vi "Turbulence_1.0.vi"() -> ()   [LabVIEW 2018]
uses:
  <instrlib>/Quantum Composers 9000 Series 2.08/Quantum Composers 9000 Series.lvlib
  <userlib>/LightField Add-in and Automation SDK/Samples/LabVIEW Automation/lightfield-automation-labview/LightField Automation.lvclass
panel:
  in  "Number of Frames":i32
  in  "Intensifier Gain":i32
  in  "Repetitive Gate Width (us)":dbl
  in  "On Chip Accumulations":i32=6
  out "Intensity Graph":dbl[][](graph)
  in  "Experiment Name":string="Experiment1"
  in  "?":bool
  in  "?":bool
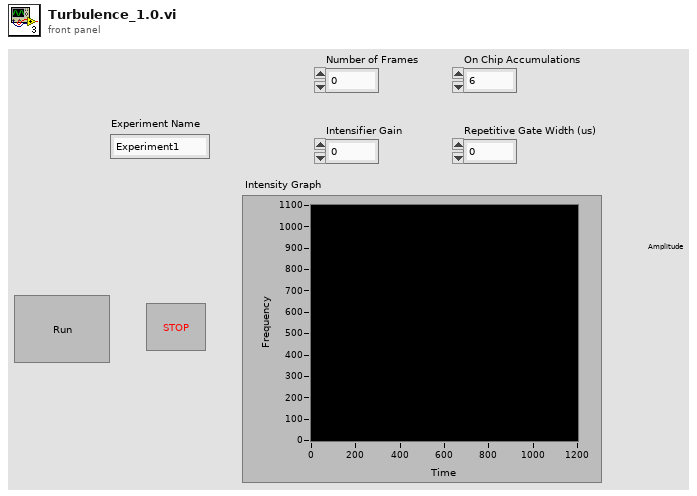
[diagram p1: front panel]
types:
  T1 = cluster{"Image":dbl[][][], "Frame Size":cluster{"F":i32, "Y":i32, "X":i32}}[]
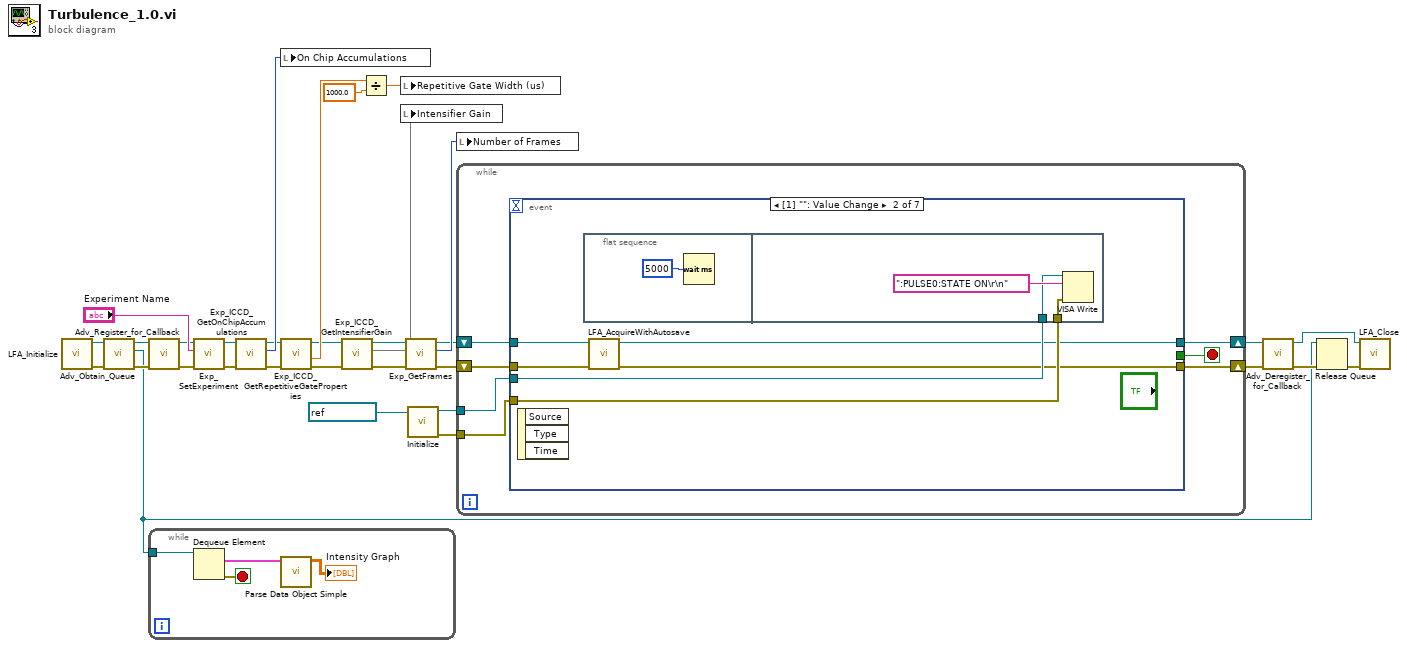
[diagram p0: block diagram]
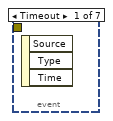
[diagram p2: hidden frame]
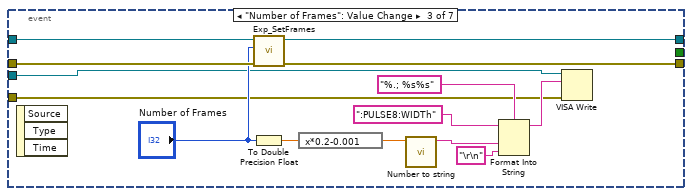
[diagram p3: hidden frame]
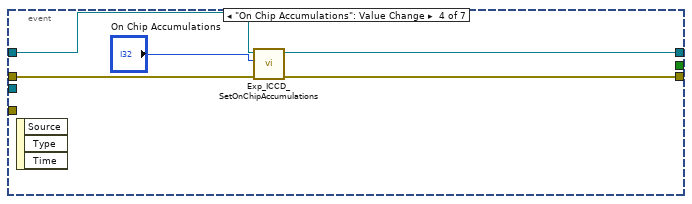
[diagram p4: hidden frame]
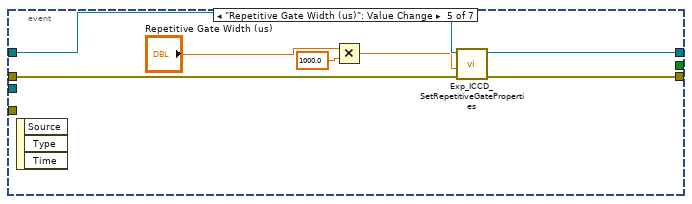
[diagram p5: hidden frame]
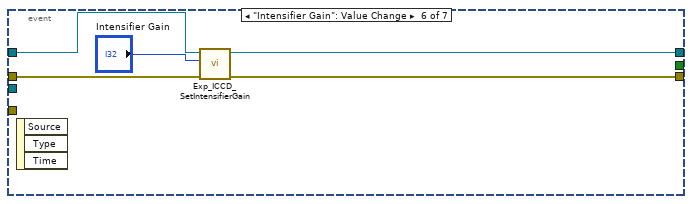
[diagram p6: hidden frame]
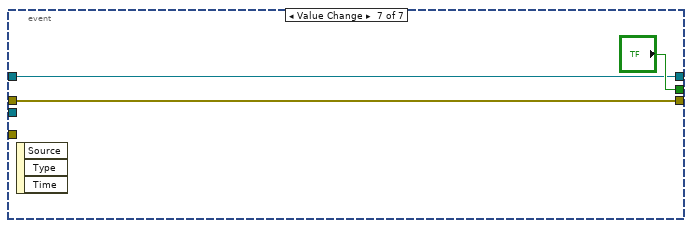
[diagram p7: hidden frame]
diagram:
  n1 = call <userlib>:"LFA_Initialize.vi"() -> ("error out"=w29:errorcluster, "LightField Automation out"=w30:refnum<class "LightField Automation.lvclass">)  [unwired: 10 in]
  n2 = call <userlib>:"Adv_Obtain_Queue.vi"("error in (no error)"=w29, "LightField Automation in"=w30) -> ("error out"=w27:errorcluster, "Queue Reference"=w16:refnum<queue>, "LightField Automation out"=w28:refnum<class "LightField Automation.lvclass">)  [unwired: 7 in]
  n3 = call <userlib>:"Adv_Register_for_Callback.vi"("error in (no error)"=w27, "LightField Automation in"=w28) -> ("error out"=w21:errorcluster, "LightField Automation out"=w22:refnum<class "LightField Automation.lvclass">)  [unwired: 8 in]
  n4 = while {
    tunnel: w16 -> [w36]
    stop <- w35 stop-if-true
    n5 = Dequeue Element(queue=w36) -> (element=w34:T1, error out=w35:errorcluster)  [unwired: 2 in, 2 out]
    n6 = call <userlib>:"Parse Data Object Simple.vi"("Data"=w34) -> ("ROI 1, Frame 1"=→"Intensity Graph":dbl[][])  [unwired: 9 in, 1 out]
  }
  n7 = call <userlib>:"Exp_SetExperiment.vi"("error in (no error)"=w21, "ExperimentName"="Experiment Name", "LightField Automation in"=w22) -> ("error out"=w17:errorcluster, "LightField Automation out"=w18:refnum<class "LightField Automation.lvclass">)  [unwired: 7 in]
  n8 = call <userlib>:"Exp_ICCD_GetOnChipAccumulations.vi"("error in (no error)"=w17, "LightField Automation in"=w18) -> ("error out"=w13:errorcluster, "On Chip Accumulations"=w15:i32, "LightField Automation out"=w14:refnum<class "LightField Automation.lvclass">)  [unwired: 7 in]
  n9 = local write "On Chip Accumulations"(w15) -> ()
  n10 = call <userlib>:"Exp_ICCD_GetRepetitiveGateProperties.vi"("error in (no error)"=w13, "LightField Automation in"=w14) -> ("error out"=w8:errorcluster, "Repetitive Gate Width (ns)"=w12:dbl, "LightField Automation out"=w9:refnum<class "LightField Automation.lvclass">)  [unwired: 6 in, 1 out]
  n11 = call <userlib>:"Exp_ICCD_GetIntensifierGain.vi"("error in (no error)"=w8, "LightField Automation in"=w9) -> ("error out"=w5:errorcluster, 2:w1, "LightField Automation out"=w6:refnum<class "LightField Automation.lvclass">)  [unwired: 6 in, 1 out]
  n12 = Divide(x=w12, y=1000.0) -> (x/y=w10:dbl)
  n13 = local write "Repetitive Gate Width (us)"(w10) -> ()
  n14 = local write "Intensifier Gain"(w1) -> ()
  n15 = call <userlib>:"Exp_GetFrames.vi"("error in (no error)"=w5, "LightField Automation in"=w6) -> ("error out"=w4:errorcluster, "Frames"=w7:i32, "LightField Automation out"=w3:refnum<class "LightField Automation.lvclass">)  [unwired: 7 in]
  n16 = call <instrlib>:"Initialize.vi"("VISA resource name"=refnum<visa-resource-name> "COM16") -> ("error out"=w31:errorcluster, "VISA resource name out"=w32:refnum<visa-resource-name>)  [unwired: 9 in]
  n17 = local write "Number of Frames"(w7) -> ()
  n18 = while {
    tunnel: w32 -> [w42]
    tunnel: w31 -> [w43]
    shift-right: [w40] -> w20
    shift-left: w3 -> [w38]
    shift-right: [w41] -> w19
    shift-left: w4 -> [w39]
    stop <- w37 stop-if-true
    n19 = event shown="[1] \"\": Value Change" {
      selector: _ -> [_ _ _ _ _ _ _]
      dyn-events: _ -> [_ _ _ _ _ _ _]
      timeout: _ -> [_ _ _ _ _ _ _]
      tunnel: w43 -> [_ w49 w57 _ _ _ _]
      tunnel: w42 -> [_ w48 w58 _ _ _ _]
      tunnel: w39 -> [_ w47 w64 w71 w78 w82 w85]
      tunnel: w38 -> [_ w46 w67 w72 w79 w83 w86]
      tunnel: [_ w45 w65 w69 w76 w80 w85] -> w41
      tunnel: [_ w44 w66 w70 w77 w81 w86] -> w40
      tunnel: [_ _ _ _ _ _ "?"] -> w37
      event Timeout {
        n20 = event-data() -> ()  [unwired: 1 in, 3 out]
      }
      event Value Change {
        n21 = event-data() -> ()  [unwired: 1 in, 3 out]
        n22 = flat-sequence {
          tunnel: w49 -> [w53]
          tunnel: w48 -> [w51]
          frame #0 {
            n23 = Wait (ms)(milliseconds to wait=5000) -> ()  [unwired: 1 out]
          }
          frame #1 {
            n24 = VISA Write(VISA resource name=w51, write buffer=":PULSE0:STATE ON\r\n" ("format string"), error in (no error)=w53) -> ()  [unwired: 3 out]
          }
        }
        n25 = call <userlib>:"LFA_AcquireWithAutosave.vi"("error in (no error)"=w47, "LightField Automation in"=w46) -> ("error out"=w45:errorcluster, "LightField Automation out"=w44:refnum<class "LightField Automation.lvclass">)  [unwired: 7 in, 1 out]
      }
      event "Number of Frames": Value Change {
        n26 = event-data() -> ()  [unwired: 1 in, 3 out]
        n27 = call <userlib>:"Exp_SetFrames.vi"("error in (no error)"=w64, "Number of Frames"="Number of Frames", "LightField Automation in"=w67) -> ("error out"=w65:errorcluster, "LightField Automation out"=w66:refnum<class "LightField Automation.lvclass">)  [unwired: 7 in]
        n28 = To Double Precision Float(number="Number of Frames") -> (double precision float=w62:dbl)
        n29 = expression code="x*0.2-0.001"(w62) -> (w56:dbl)
        n30 = call "Number to string.vi"("Numeric"=w56) -> ("Shortest String"=w55:string)  [unwired: 10 in]
        n31 = Format Into String(format string="%.; %s%s", initial string=":PULSE8:WIDTh" ("format string"), w55, "\r\n" ("format string")) -> (resulting string=w59:string)  [unwired: 1 in, 1 out]
        n32 = VISA Write(VISA resource name=w58, write buffer=w59, error in (no error)=w57) -> ()  [unwired: 3 out]
      }
      event "On Chip Accumulations": Value Change {
        n33 = event-data() -> ()  [unwired: 1 in, 3 out]
        n34 = call <userlib>:"Exp_ICCD_SetOnChipAccumulations.vi"("error in (no error)"=w71, "On Chip Accumulations"="On Chip Accumulations", "LightField Automation in"=w72) -> ("error out"=w69:errorcluster, "LightField Automation out"=w70:refnum<class "LightField Automation.lvclass">)  [unwired: 7 in]
      }
      event "Repetitive Gate Width (us)": Value Change {
        n35 = event-data() -> ()  [unwired: 1 in, 3 out]
        n36 = Multiply(x="Repetitive Gate Width (us)", y=1000.0) -> (x*y=w73:dbl)
        n37 = call <userlib>:"Exp_ICCD_SetRepetitiveGateProperties.vi"("error in (no error)"=w78, "Repetitive Gate Width (ns)"=w73, "LightField Automation in"=w79) -> ("error out"=w76:errorcluster, "LightField Automation out"=w77:refnum<class "LightField Automation.lvclass">)  [unwired: 7 in]
      }
      event "Intensifier Gain": Value Change {
        n38 = event-data() -> ()  [unwired: 1 in, 3 out]
        n39 = call <userlib>:"Exp_ICCD_SetIntensifierGain.vi"("error in (no error)"=w82, "Intensifier Gain"="Intensifier Gain", "LightField Automation in"=w83) -> ("error out"=w80:errorcluster, "LightField Automation out"=w81:refnum<class "LightField Automation.lvclass">)  [unwired: 7 in]
      }
      event Value Change {
        n40 = event-data() -> ()  [unwired: 1 in, 3 out]
      }
    }
  }
  n41 = call <userlib>:"Adv_Deregister_for_Callback.vi"("error in (no error)"=w19, "LightField Automation in"=w20) -> ("error out"=w26:errorcluster, "LightField Automation out"=w24:refnum<class "LightField Automation.lvclass">)  [unwired: 8 in]
  n42 = Release Queue(queue=w16, error in (no error)=w26) -> (error out=w25:errorcluster)  [unwired: 1 in, 2 out]
  n43 = call <userlib>:"LFA_Close.vi"("error in (no error)"=w25, "LightField Automation in"=w24) -> ()  [unwired: 8 in, 2 out]
